vi "launch_vi_transition.vi"(8 "error in (no error)":errorcluster, 10 "data":T1={"current_state"=enum."<automatic_state>", "previous_state"=enum."<automatic_state>", "criteria"=variant, "data"=variant, "recipe_data"=variant(dbl 0.6680663352984317), "index"=-1, "step"="", "steps"=variant}, 11 "vi_reference":variant) -> (0 "error out":errorcluster, 1 "index out":i32, 3 "recipe_data out":variant)   [LabVIEW 2015, in "lv-recipe-machine.lvlib"]
uses:
  lv-recipe-machine.lvlib
  _controls/automatic_vi_variant_data.ctl
  public/_controls/automatic_state.ctl
  public/_controls/error.ctl
  public/_controls/vi_reference_type.ctl
  public/_controls/vi_reference_transition.ctl
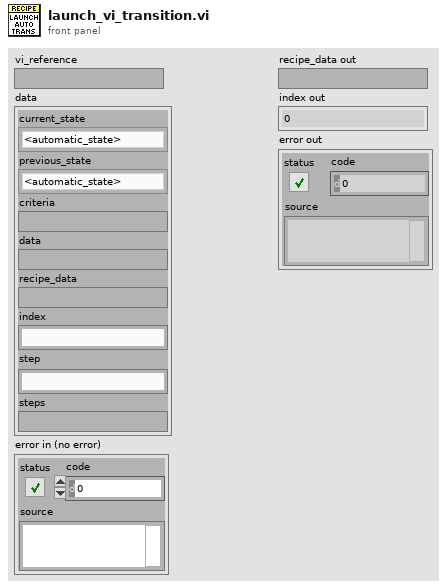
[diagram p1: front panel]
types:
  T1 = typedef "lv-recipe-machine.lvlib/automatic_vi_variant_data.ctl" = cluster{"current_state":T2, "previous_state":T2, "criteria":variant, "data":variant, "recipe_data":variant, "index":i32, "step":string, "steps":variant}
  T2 = typedef "lv-recipe-machine.lvlib/automatic_state.ctl" = enum16{"<automatic_state>", "failed", "idle", "running", "paused", "stopped", "<null>"}
  T3 = typedef "lv-recipe-machine.lvlib/error.ctl" = enum16{"<error>", "bad_command", "command_queue_timeout", "stop_notifier_timeout", "die_command_timeout", "not_in_manual_mode", "not_in_automatic_mode", "not_in_automatic_idle", "not_in_automatic_running", "not_in_automatic_paused", "automatic_step_not_found", "manual_action_not_found", "automatic_not_transition_vi", "transition_step_not_found", "unsupported_vi_type", "<null>"}
  T4 = typedef "lv-recipe-machine.lvlib/vi_reference_type.ctl" = enum16{"<vi_reference_type>", "manual_action", "auto_step", "auto_criteria", "auto_transition", "auto_launcher", "<null>"}
  T5 = typedef "lv-recipe-machine.lvlib/vi_reference_transition.ctl" = refnum<vi>
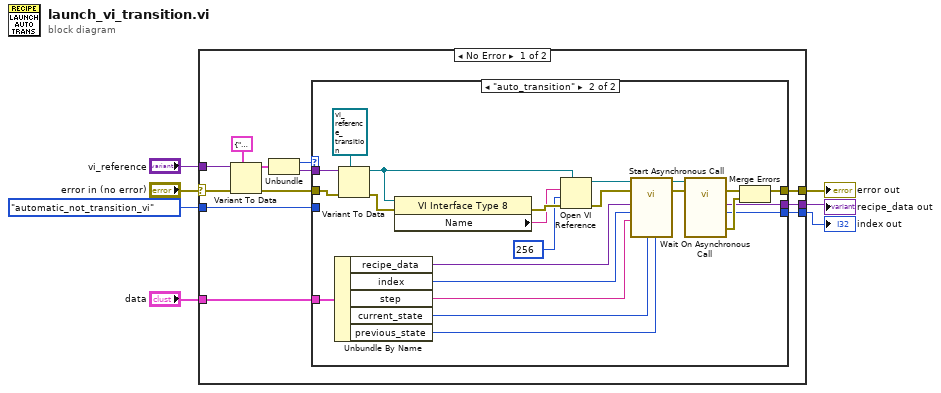
[diagram p0: block diagram]
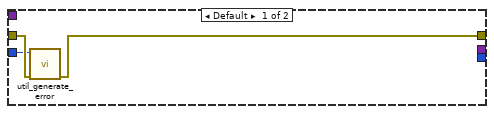
[diagram p2: hidden frame]
diagram:
  n1 = case shown="No Error" "error in (no error)" {
    selector: "error in (no error)" -> [w17 w46]
    tunnel: [w13 w46] -> w6
    tunnel: "vi_reference" -> [w18 _]
    tunnel: [w12 _] -> w4
    tunnel: [w11 _] -> w3
    tunnel: error."automatic_not_transition_vi" ("error") -> [w9 _]
    tunnel: "data" -> [w8 _]
    frame No Error {
      n2 = Variant To Data(error in=w17, type=cluster{"vi_reference_type":T4, variant} {"vi_reference_type"=enum."<vi_reference_type>", variant}, Variant=w18) -> (data=w16:cluster{"vi_reference_type":T4, variant}, error out=w15:errorcluster)
      n3 = Unbundle(w16) -> ("vi_reference_type"=w10:T4, w14:variant)
      n4 = case shown="\"auto_transition\"" w10 {
        tunnel: w15 -> [w22 w45]
        tunnel: w14 -> [_ w44]
        tunnel: [w21 w33] -> w13
        tunnel: [_ w30] -> w12
        tunnel: [_ w29] -> w11
        tunnel: w9 -> [w20 _]
        tunnel: w8 -> [_ w28]
        frame Default {
          n5 = call "util_generate_error.vi"("error in (no error)"=w22, "error"=w20) -> ("error out"=w21:errorcluster)  [unwired: 9 in]
        }
        frame "auto_transition" {
          n6 = Unbundle By Name(w28) -> ("recipe_data"=w27:variant, "index"=w24:i32, "step"=w23:string, "current_state"=w25:T2, "previous_state"=w26:T2)
          n7 = Variant To Data(error in=w45, type=T5 refnum ("vi_reference_transition"), Variant=w44) -> (data=w37:T5, error out=w31:errorcluster)
          n8 = property class="VI Interface Type 8"(reference=w37, error in=w31) -> (error out=w43:errorcluster, "Name"=w40:string)  [unwired: 1 out]
          n9 = Open VI Reference(type specifier VI Refnum (for type only)=w37, vi path=w40, options=256, error in (no error)=w43) -> (vi reference=w39:T5, error out=w41:errorcluster)  [unwired: 2 in]
          n10 = call-by-ref "Start Asynchronous Call"(reference=w39, error in=w41, "previous_state"=w26, "current_state"=w25, "step"=w23, "index in"=w24, "recipe_data in"=w27) -> (reference out=w34:T5, error out=w36:errorcluster)  [unwired: 4 in, 3 out]
          n11 = call-by-ref "Wait On Asynchronous Call"(reference=w34, error in=w36) -> (error out=w35:errorcluster, 0:"error out"=w32:errorcluster, "index out"=w29:i32, "recipe_data out"=w30:variant)  [unwired: 9 in, 1 out]
          n12 = Merge Errors(w35, w32) -> (w33:errorcluster)
        }
      }
    }
    frame Error {
    }
  }
  "error out" <- w6
  "recipe_data out" <- w4
  "index out" <- w3
